vi "Find Outline.vi"(6 "Mask Info":i8[][](array[numeric]), 7 "Data":u8[][](array[numeric]), 8 "error in (no error)":errorcluster, 9 "Starting X (left)":i32, 10 "Starting Y (top)":i32, 11 "Outline in":refnum<class "Outline.lvclass">) -> (0 "error out":errorcluster, 3 "Outline out":refnum<class "Outline.lvclass">, 4 "Mask Info out":i8[][](array[numeric]))   [LabVIEW 2013, in "Outline.lvclass"]
uses:
  Outline.lvclass
  Outline.lvclass/Outline.ctl
  <vilib>/vision/NI_Vision_Development_Module.lvlib
panel:
  out "Mask Info out 2":i8[][](array[numeric])
  out "Image 3":T1(plugin-control)
  out "Image 2":T1(plugin-control)
  in  "Maximum number of points":i32=1000
  out "XY Graph":cluster{"X Values":i32[], "Y Values":i32[]}(graph)
  out "Y Values":i32[](array[numeric])
  out "X Values":i32[](array[numeric])
  # "Top first, then left"
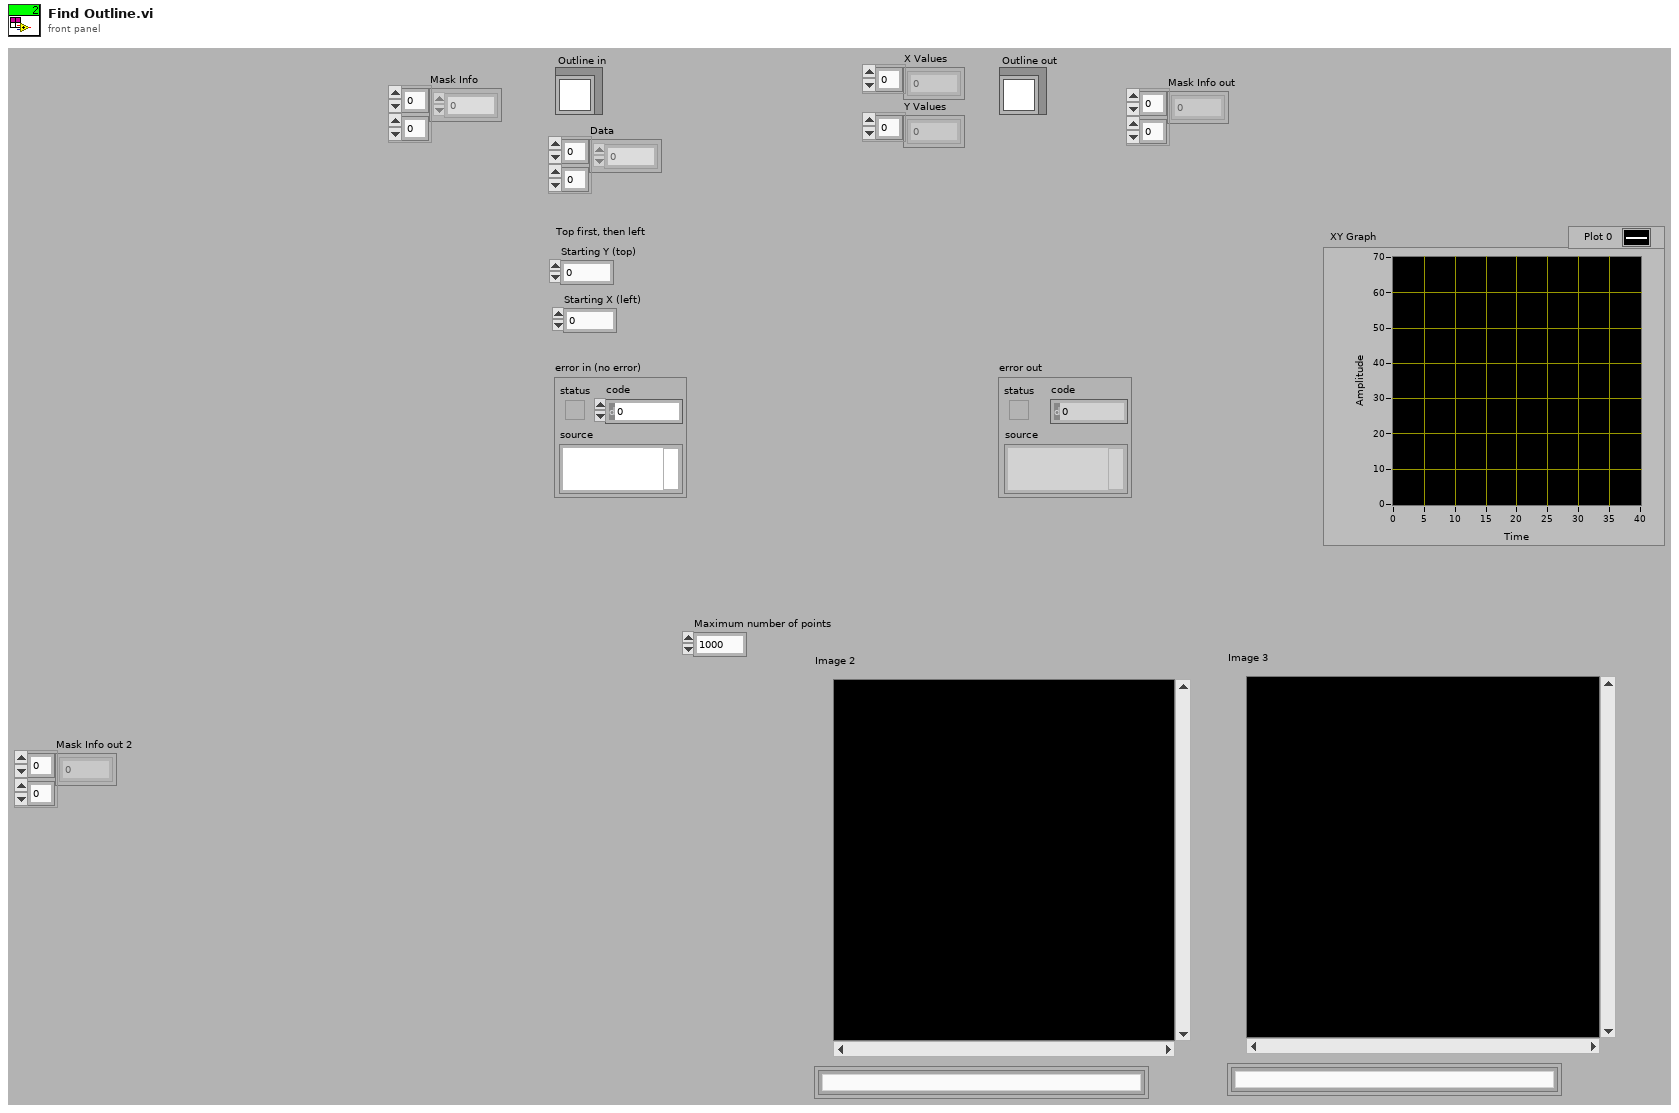
[diagram p1: front panel]
types:
  T1 = typedef "IMAQ Image.ctl" = refnum<image>
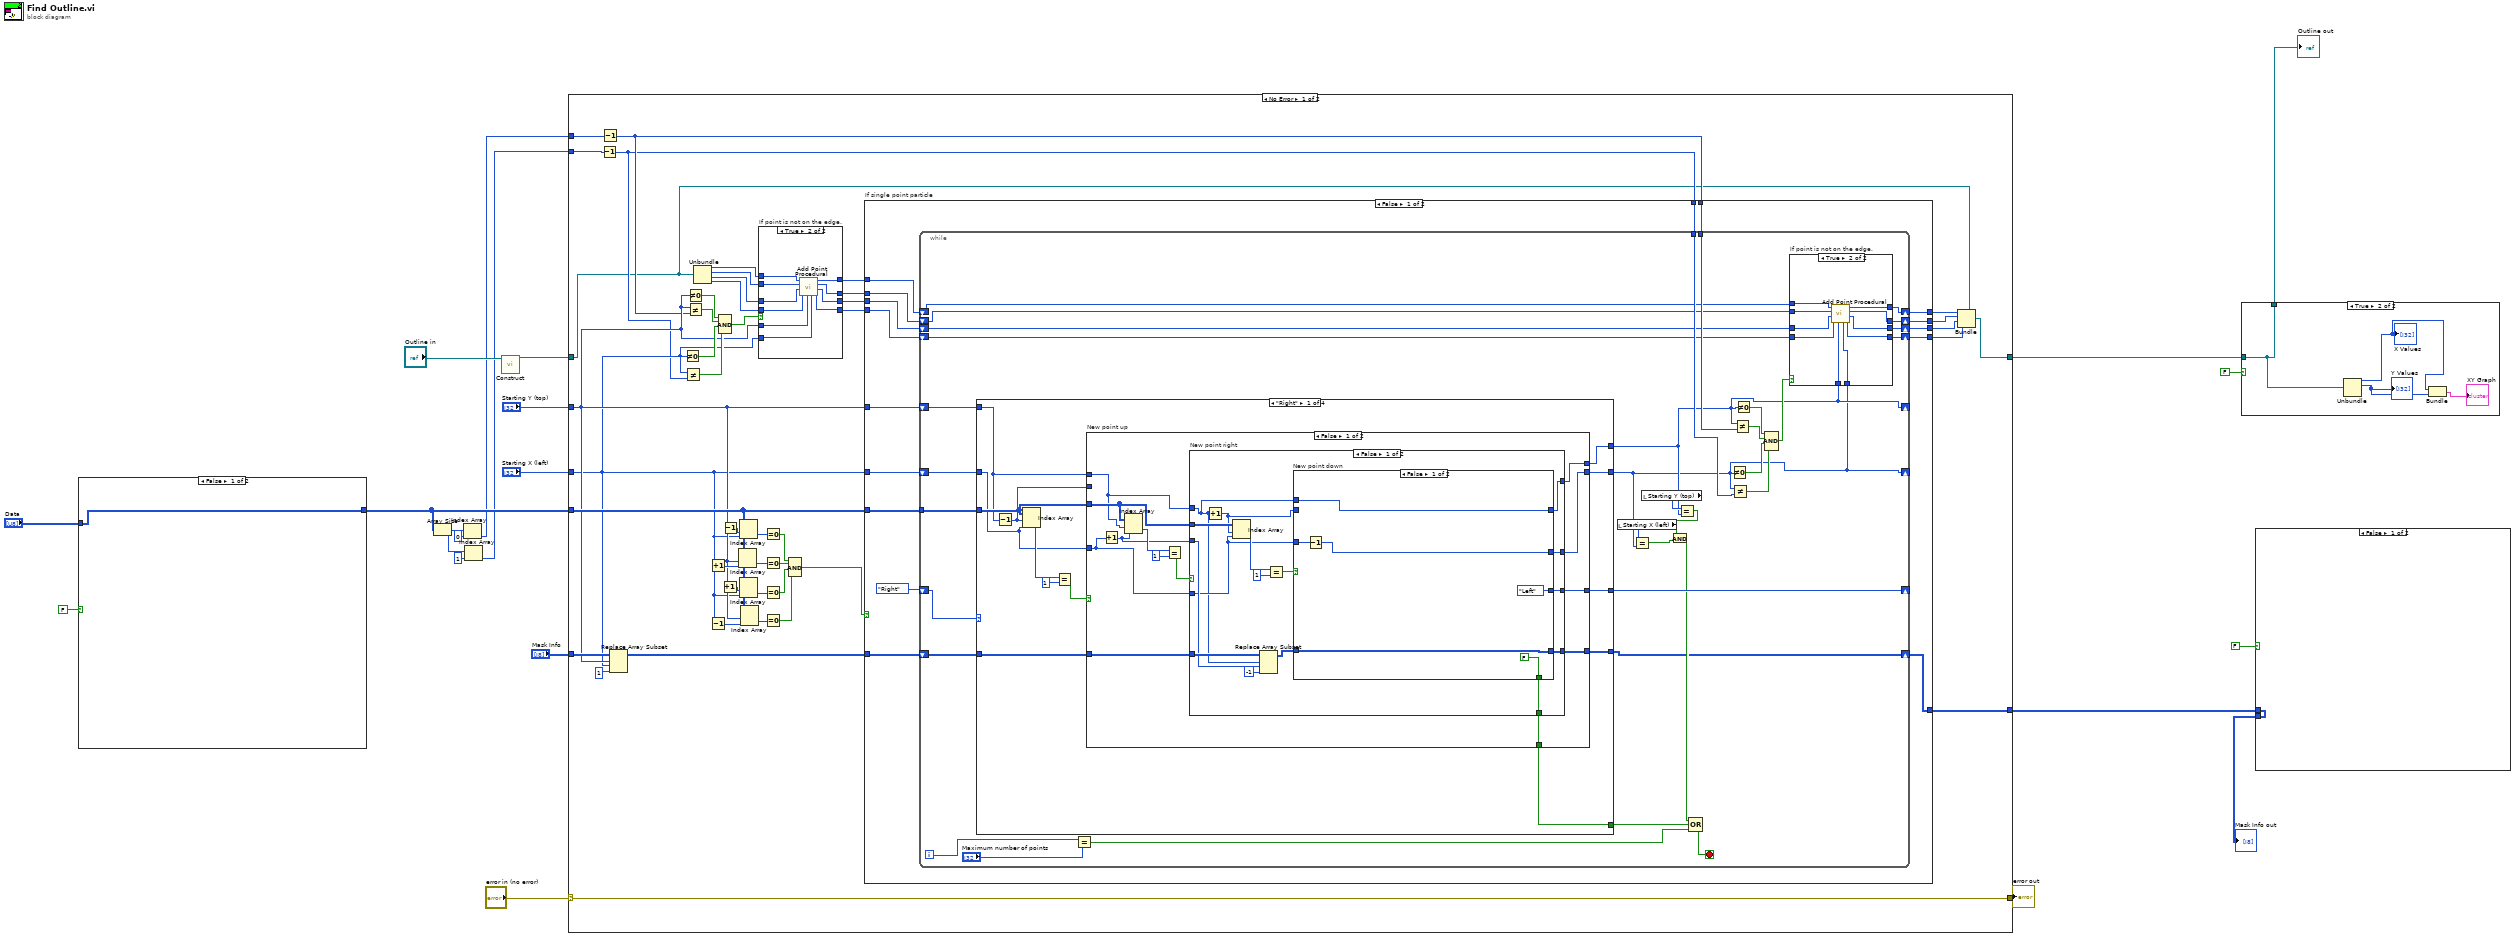
[diagram p0: block diagram]
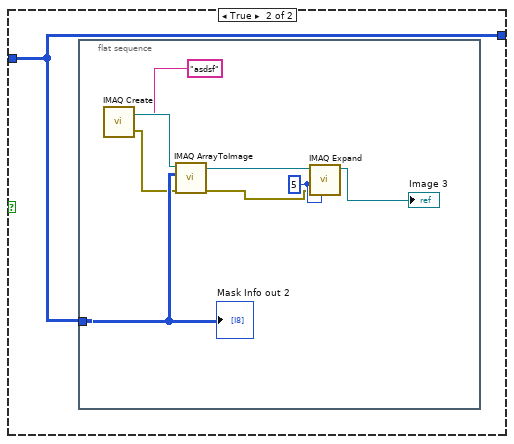
[diagram p2: hidden frame]
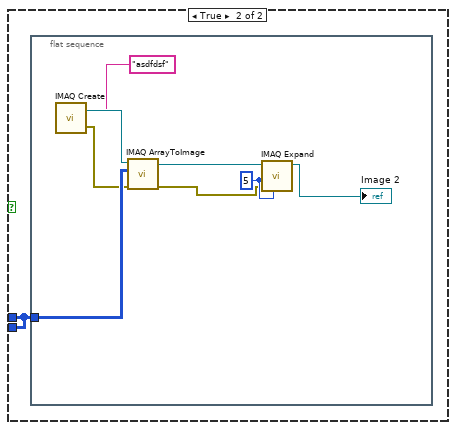
[diagram p3: hidden frame]
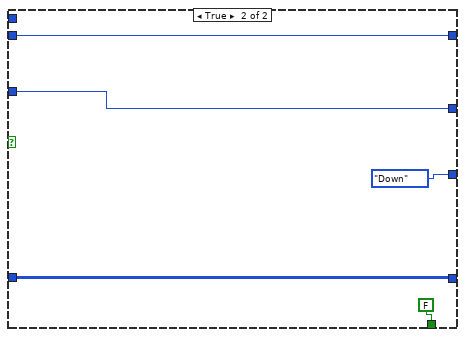
[diagram p7: hidden frame]
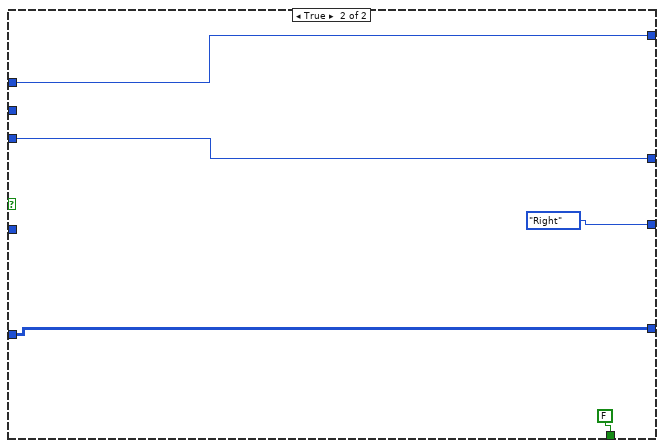
[diagram p8: hidden frame]
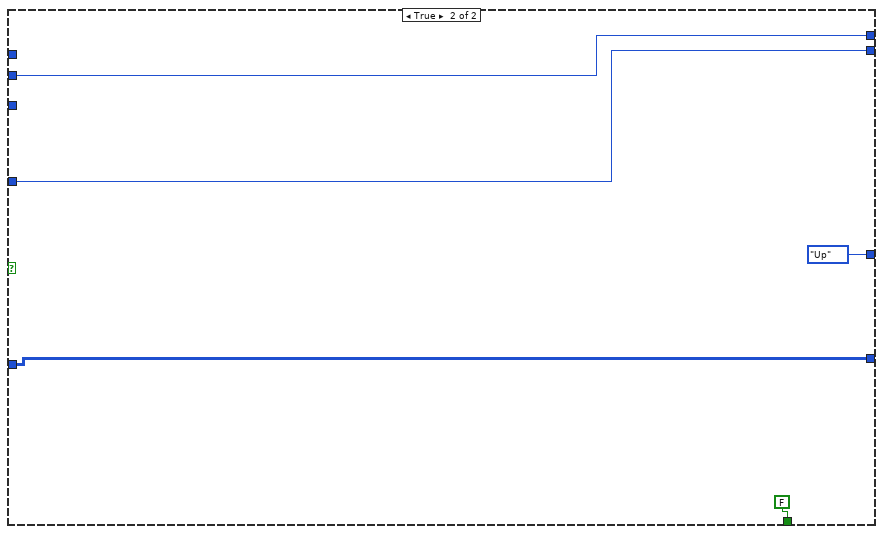
[diagram p9: hidden frame]
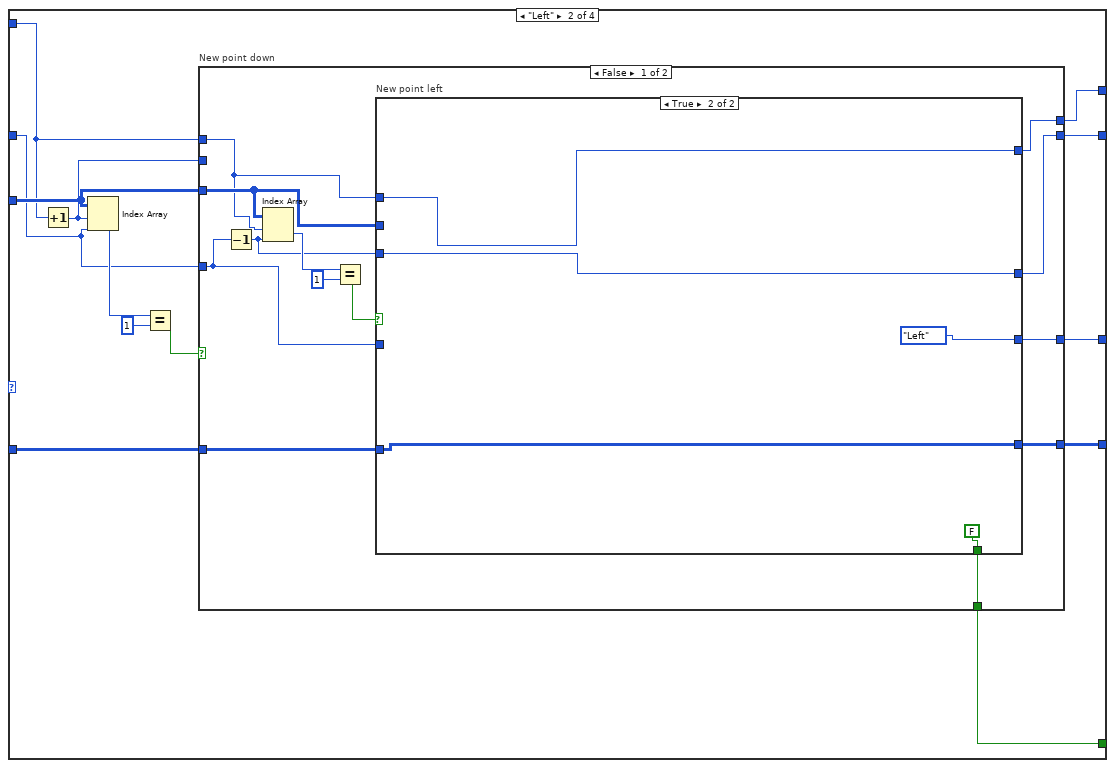
[diagram p10: hidden frame]
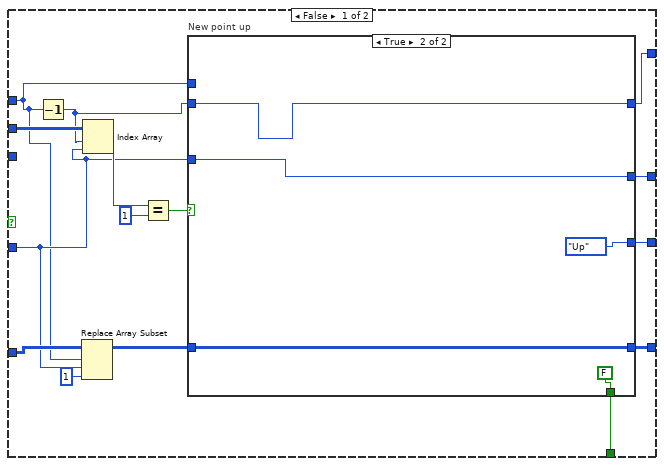
[diagram p11: hidden frame]
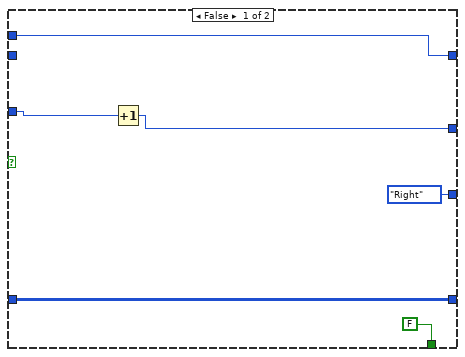
[diagram p12: hidden frame]
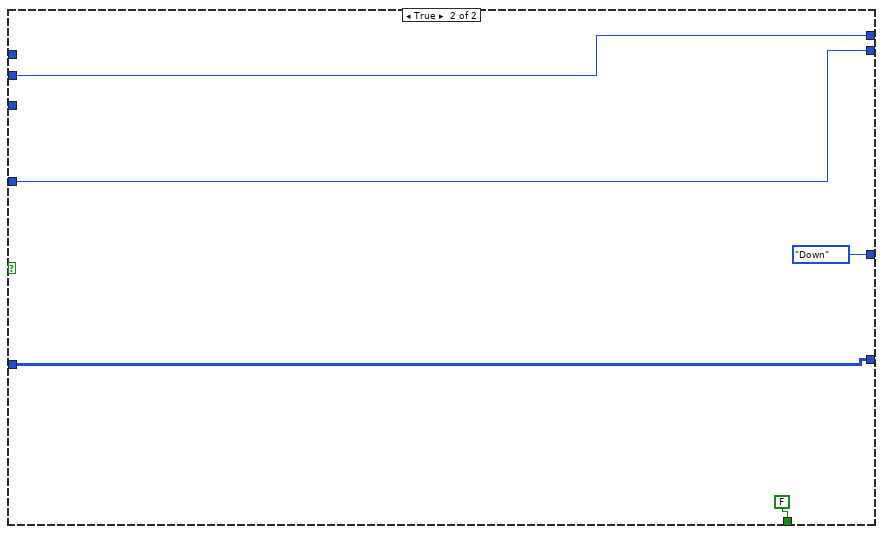
[diagram p13: hidden frame]
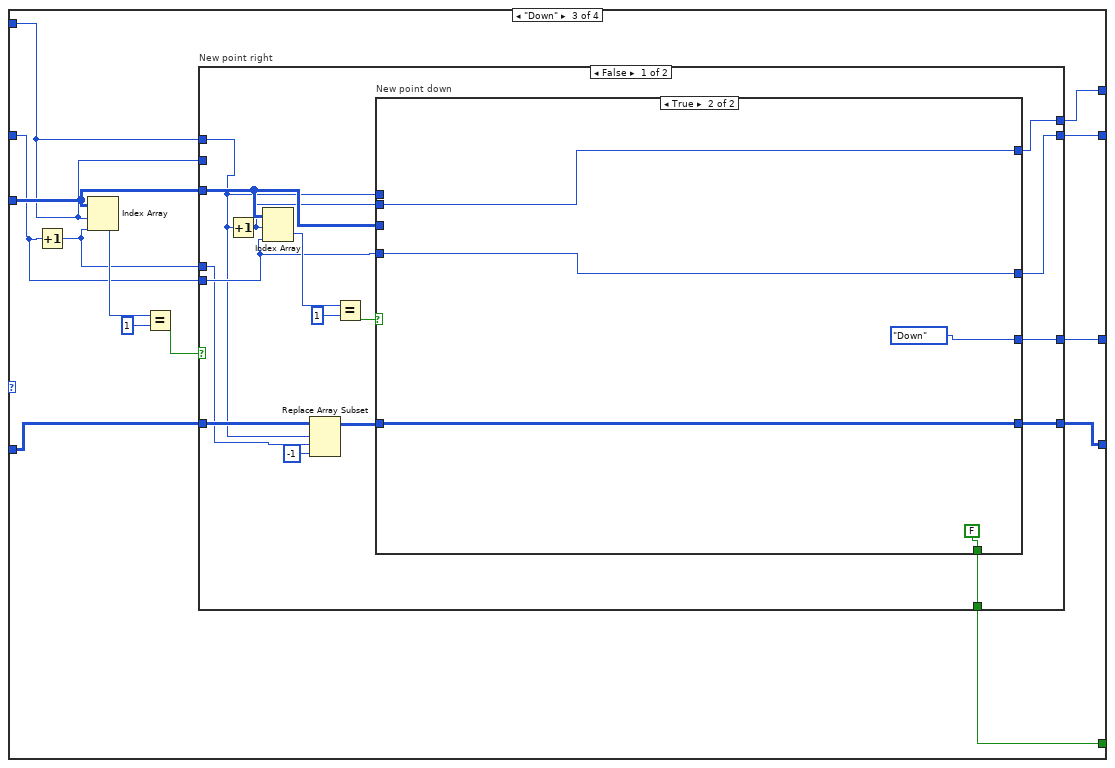
[diagram p14: hidden frame]
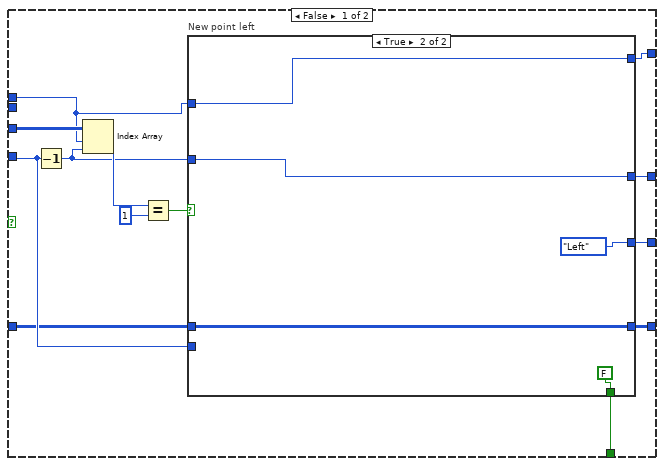
[diagram p15: hidden frame]
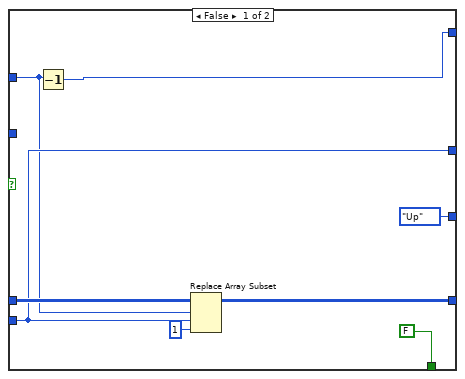
[diagram p16: hidden frame]
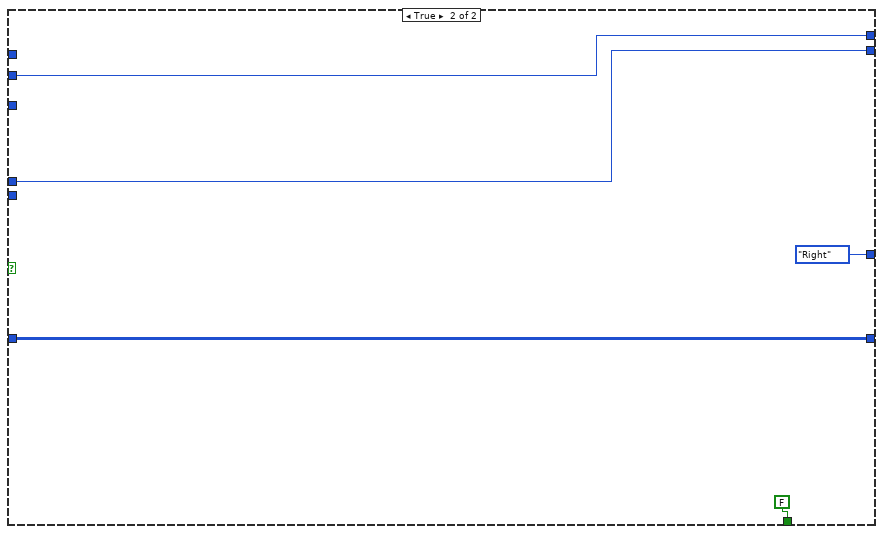
[diagram p17: hidden frame]
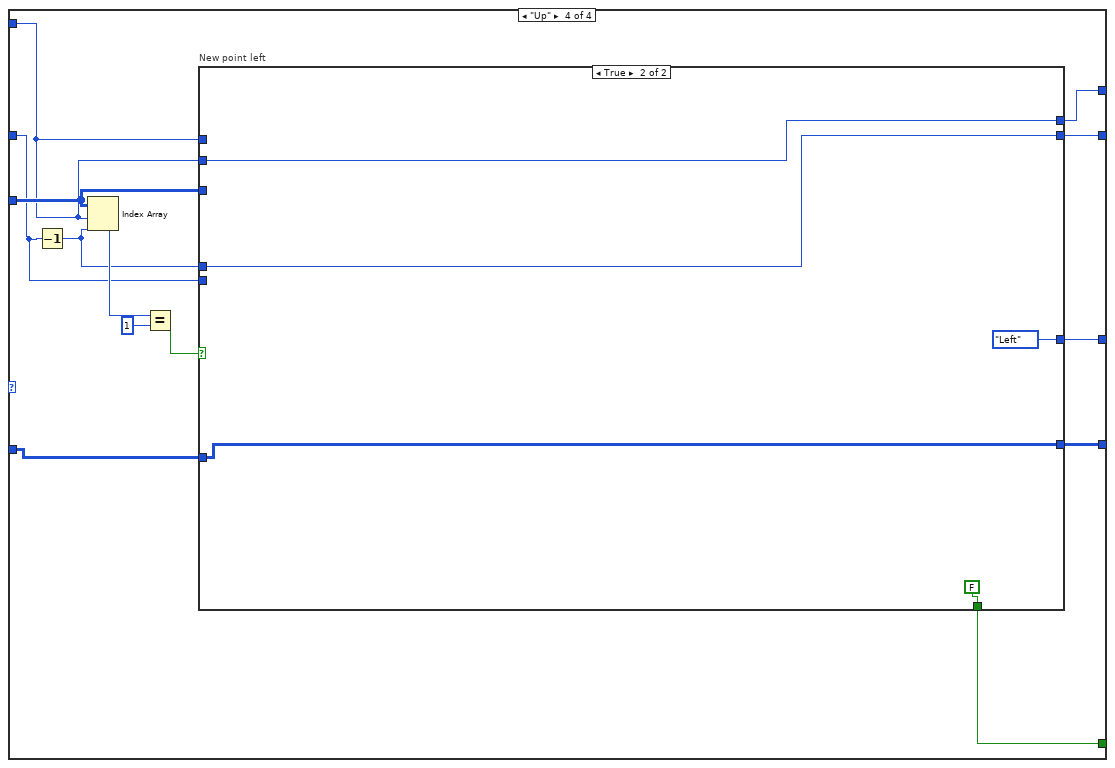
[diagram p18: hidden frame]
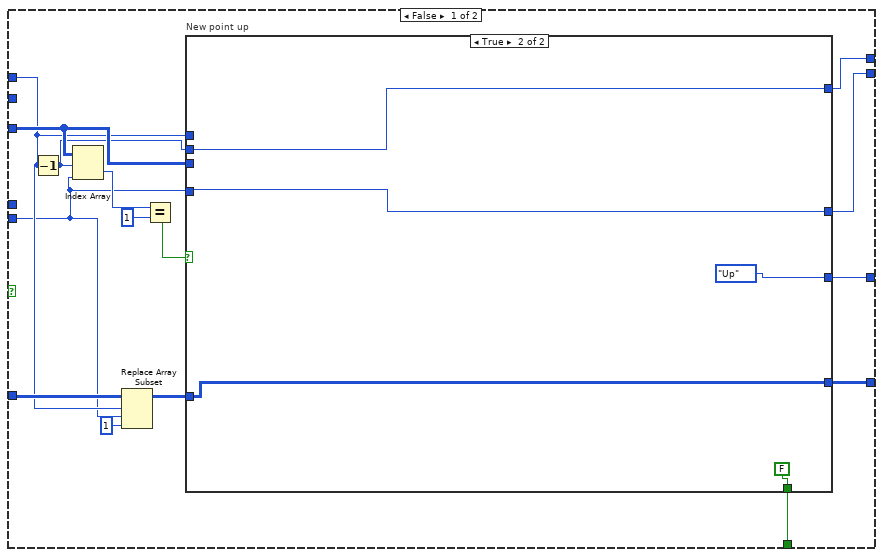
[diagram p19: hidden frame]
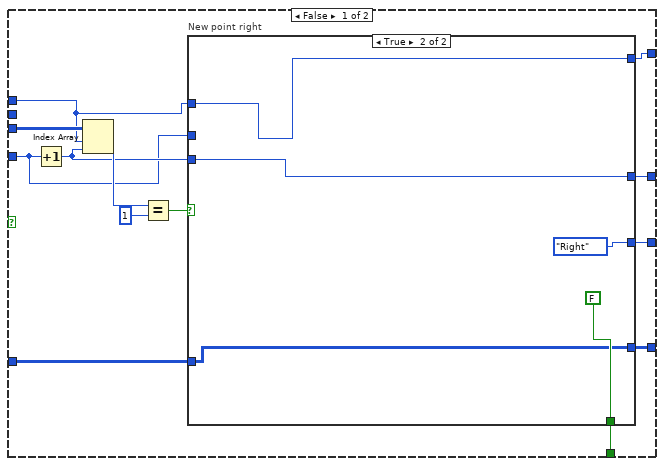
[diagram p20: hidden frame]
diagram:
  n1 = case shown="False" FALSE {
    tunnel: [w22 w23] -> w3
    tunnel: "Data" -> [w22 w23]
    frame False {
    }
    frame True {
      n2 = flat-sequence {
        tunnel: w23 -> [w30]
        frame #0 {
          w31 = 5 ("X Duplication Step")
          n3 = call "IMAQ Create"("Image Name"="asdsf") -> ("New Image"=w25:T1, "error out"=w26:errorcluster)  [unwired: 4 in]
          n4 = call "IMAQ ArrayToImage"("error in (no error)"=w26, "Image Pixels (U8)"=w30, "Image"=w25) -> ("error out"=w28:errorcluster, "Image Out"=w29:T1)  [unwired: 7 in]
          n5 = call "IMAQ Expand"("Y Duplication Step"=w31, "error in (no error)"=w28, "X Duplication Step"=w31, "Image Src"=w29) -> ("Image Dst Out"=→"Image 3":T1)  [unwired: 6 in, 1 out]
          "Mask Info out 2" <- w30
        }
      }
    }
  }
  n6 = Array Size(array=w3) -> (size(s)=w7:i32[])
  n7 = Index Array(array=w7, index=0) -> (element=w2:i32)
  n8 = Index Array(array=w7, index=1) -> (element=w1:i32)
  n9 = call-dynamic "Construct.vi"("Outline in"="Outline in") -> ("Outline out"=w17:refnum<class "Outline.lvclass">)  [unwired: 9 in, 1 out]
  n10 = case shown="No Error" "error in (no error)" {
    selector: "error in (no error)" -> [w75 w420]
    tunnel: [w75 w420] -> w21
    tunnel: [w32 w419] -> w20
    tunnel: w17 -> [w37 w419]
    tunnel: "Starting Y (top)" -> [w51 _]
    tunnel: "Starting X (left)" -> [w50 _]
    tunnel: w3 -> [w69 _]
    tunnel: "Mask Info" -> [w73 w418]
    tunnel: [w74 w418] -> w9
    tunnel: w2 -> [w41 _]
    tunnel: w1 -> [w39 _]
    frame No Error {
      n11 = Decrement(x=w39) -> (x-1=w38:i32)
      n12 = Decrement(x=w41) -> (x-1=w40:i32)
      n13 = Replace Array Subset(array=w73, new element=i8 1 ("new element/subarray"), index (row)=w51, index (col)=w50) -> (w72:i8[][])
      n14 = Not Equal To 0?(x=w50) -> (x != 0?=w54:bool)
      n15 = Not Equal?(x=w50, y=w38) -> (x != y?=w55:bool)
      n16 = Not Equal To 0?(x=w51) -> (x != 0?=w52:bool)
      n17 = Not Equal?(x=w51, y=w40) -> (x != y?=w53:bool)
      n18 = Unbundle(w37) -> (w49:i32[], w46:i32[], w47:i32, w48:i32)
      n19 = Increment(x=w50) -> (x+1=w68:i32)
      n20 = Decrement(x=w50) -> (x-1=w66:i32)
      n21 = Compound Arithmetic op=AND(w52, w53, w54, w55) -> (w56:bool)
      n22 = Increment(x=w51) -> (x+1=w67:i32)
      n23 = Decrement(x=w51) -> (x-1=w70:i32)
      n24 = Index Array(array=w69, index (row)=w51, index (col)=w68) -> (element=w64:u8)
      n25 = Index Array(array=w69, index (row)=w70, index (col)=w50) -> (element=w65:u8)
      n26 = Index Array(array=w69, index (row)=w67, index (col)=w50) -> (element=w63:u8)
      n27 = Index Array(array=w69, index (row)=w51, index (col)=w66) -> (element=w62:u8)
      n28 = case "If point is not on the edge." shown="True" w56 {
        tunnel: w51 -> [_ w89]
        tunnel: w50 -> [_ w88]
        tunnel: w49 -> [w79 w87]
        tunnel: w46 -> [w78 w86]
        tunnel: w47 -> [w77 w85]
        tunnel: w48 -> [w76 w84]
        tunnel: [w79 w83] -> w45
        tunnel: [w78 w82] -> w44
        tunnel: [w77 w81] -> w43
        tunnel: [w76 w80] -> w42
        frame False {
        }
        frame True {
          n29 = call "Add Point Procedural.vi"("New X"=w88, "New Y"=w89, "Memory allocated in"=w84, "Number of points in"=w85, "Y Values in"=w86, "X Values in"=w87) -> ("Memory allocated out"=w80:i32, "Number of Points out"=w81:i32, "Y Values out"=w82:i32[], "X Values out"=w83:i32[])  [unwired: 2 in]
        }
      }
      n30 = Equal To 0?(x=w65) -> (x = 0?=w61:bool)
      n31 = Equal To 0?(x=w64) -> (x = 0?=w60:bool)
      n32 = Equal To 0?(x=w63) -> (x = 0?=w59:bool)
      n33 = Equal To 0?(x=w62) -> (x = 0?=w58:bool)
      n34 = Compound Arithmetic op=AND(w61, w60, w59, w58) -> (w57:bool)
      n35 = case "If single point particle" shown="False" w57 {
        tunnel: [w104 w412] -> w74
        tunnel: w72 -> [w103 w417]
        tunnel: w69 -> [w102 _]
        tunnel: w50 -> [w101 w415]
        tunnel: w51 -> [w100 w416]
        tunnel: w40 -> [w99 _]
        tunnel: w38 -> [w98 _]
        tunnel: w45 -> [w97 w411]
        tunnel: w44 -> [w96 w410]
        tunnel: w43 -> [w95 w409]
        tunnel: w42 -> [w94 w408]
        tunnel: [w93 w411] -> w36
        tunnel: [w92 w410] -> w35
        tunnel: [w91 w409] -> w34
        tunnel: [w90 w408] -> w33
        frame False {
          n36 = while {
            shift-right: [w115] -> _
            shift-left: w100 -> [w138]
            shift-right: [w114] -> _
            shift-left: w101 -> [w137]
            shift-right: [w135] -> _
            shift-left: enum16{"Up", "Left", "Down", "Right"}."Right" ("Enum") -> [w139]
            tunnel: w102 -> [w136]
            shift-right: [w123] -> w104
            shift-left: w103 -> [w124]
            tunnel: w99 -> [w122]
            tunnel: w98 -> [w121]
            shift-right: [w109] -> w93
            shift-left: w97 -> [w113]
            shift-right: [w108] -> w92
            shift-left: w96 -> [w112]
            shift-right: [w107] -> w91
            shift-left: w95 -> [w111]
            shift-right: [w106] -> w90
            shift-left: w94 -> [w110]
            i -> [w127]
            stop <- w128 stop-if-true
            n37 = case shown="\"Right\"" w139 {
              tunnel: w138 -> [w156 w219 w283 w348]
              tunnel: w137 -> [w157 w220 w282 w347]
              tunnel: w136 -> [w160 w223 w285 w350]
              tunnel: [w166 w229 w291 w356] -> w135
              tunnel: [w165 w228 w290 w355] -> w115
              tunnel: [w164 w227 w289 w354] -> w114
              tunnel: [w159 w222 w284 w349] -> w130
              tunnel: w124 -> [w155 w218 w280 w345]
              tunnel: [w154 w217 w279 w344] -> w123
              frame "Right" {
                n38 = Decrement(x=w156) -> (x-1=w158:i32)
                n39 = Index Array(array=w160, index (row)=w158, index (col)=w157) -> (element=w163:u8)
                n40 = Equal?(x=w163, y=u8 1) -> (x = y?=w161:bool)
                n41 = case "New point up" shown="False" w161 {
                  tunnel: [w176 enum16{"Up", "Left", "Down", "Right"}."Up" ("Enum")] -> w166
                  tunnel: w158 -> [_ w214]
                  tunnel: w157 -> [w169 w215]
                  tunnel: [w175 w214] -> w165
                  tunnel: [w174 w215] -> w164
                  tunnel: w160 -> [w173 _]
                  tunnel: [w172 FALSE] -> w159
                  tunnel: w156 -> [w171 _]
                  tunnel: w155 -> [w168 w212]
                  tunnel: [w167 w212] -> w154
                  frame False {
                    n42 = Increment(x=w169) -> (x+1=w170:i32)
                    n43 = Index Array(array=w173, index (row)=w171, index (col)=w170) -> (element=w177:u8)
                    n44 = Equal?(x=w177, y=u8 1) -> (x = y?=w178:bool)
                    n45 = case "New point right" shown="False" w178 {
                      tunnel: w171 -> [w180 w210]
                      tunnel: w170 -> [w182 w209]
                      tunnel: [w195 enum16{"Up", "Left", "Down", "Right"}."Right" ("Enum")] -> w176
                      tunnel: [w189 w210] -> w175
                      tunnel: [w188 w209] -> w174
                      tunnel: w173 -> [w194 _]
                      tunnel: [w190 FALSE] -> w172
                      tunnel: w169 -> [w181 _]
                      tunnel: w168 -> [w186 w207]
                      tunnel: [w184 w207] -> w167
                      frame False {
                        n46 = Increment(x=w180) -> (x+1=w183:i32)
                        n47 = Index Array(array=w194, index (row)=w183, index (col)=w181) -> (element=w192:u8)
                        n48 = Replace Array Subset(array=w186, new element=i8 -1 ("new element/subarray"), index (row)=w180, index (col)=w182) -> (w185:i8[][])
                        n49 = Equal?(x=w192, y=u8 1) -> (x = y?=w191:bool)
                        n50 = case "New point down" shown="False" w191 {
                          tunnel: [enum16{"Up", "Left", "Down", "Right"}."Left" ("Enum") enum16{"Up", "Left", "Down", "Right"}."Down" ("Enum")] -> w195
                          tunnel: w183 -> [_ w204]
                          tunnel: w181 -> [w197 w203]
                          tunnel: [FALSE FALSE] -> w190
                          tunnel: [w198 w204] -> w189
                          tunnel: [w196 w203] -> w188
                          tunnel: [w199 w202] -> w184
                          tunnel: w185 -> [w199 w202]
                          tunnel: w180 -> [w198 _]
                          frame False {
                            n51 = Decrement(x=w197) -> (x-1=w196:i32)
                          }
                          frame True {
                          }
                        }
                      }
                      frame True {
                      }
                    }
                  }
                  frame True {
                  }
                }
              }
              frame "Left" {
                n52 = Increment(x=w219) -> (x+1=w221:i32)
                n53 = Index Array(array=w223, index (row)=w221, index (col)=w220) -> (element=w226:u8)
                n54 = Equal?(x=w226, y=u8 1) -> (x = y?=w224:bool)
                n55 = case "New point down" shown="False" w224 {
                  tunnel: [w239 enum16{"Up", "Left", "Down", "Right"}."Down" ("Enum")] -> w229
                  tunnel: w221 -> [_ w275]
                  tunnel: w220 -> [w232 w274]
                  tunnel: [w238 w275] -> w228
                  tunnel: [w237 w274] -> w227
                  tunnel: w223 -> [w236 _]
                  tunnel: [w235 FALSE] -> w222
                  tunnel: w219 -> [w234 _]
                  tunnel: w218 -> [w231 w276]
                  tunnel: [w230 w276] -> w217
                  frame False {
                    n56 = Decrement(x=w232) -> (x-1=w233:i32)
                    n57 = Index Array(array=w236, index (row)=w234, index (col)=w233) -> (element=w240:u8)
                    n58 = Equal?(x=w240, y=u8 1) -> (x = y?=w241:bool)
                    n59 = case "New point left" shown="True" w241 {
                      tunnel: w234 -> [w243 w272]
                      tunnel: w233 -> [_ w271]
                      tunnel: [w257 enum16{"Up", "Left", "Down", "Right"}."Left" ("Enum")] -> w239
                      tunnel: [w251 w272] -> w238
                      tunnel: [w250 w271] -> w237
                      tunnel: w236 -> [w256 _]
                      tunnel: [w252 FALSE] -> w235
                      tunnel: w232 -> [w247 _]
                      tunnel: w231 -> [w248 w269]
                      tunnel: [w244 w269] -> w230
                      frame False {
                        n60 = Decrement(x=w243) -> (x-1=w249:i32)
                        n61 = Replace Array Subset(array=w248, new element=i8 1 ("new element/subarray"), index (row)=w243, index (col)=w247) -> (w245:i8[][])
                        n62 = Index Array(array=w256, index (row)=w249, index (col)=w247) -> (element=w254:u8)
                        n63 = Equal?(x=w254, y=u8 1) -> (x = y?=w253:bool)
                        n64 = case "New point up" shown="True" w253 {
                          tunnel: [enum16{"Up", "Left", "Down", "Right"}."Right" ("Enum") enum16{"Up", "Left", "Down", "Right"}."Up" ("Enum")] -> w257
                          tunnel: w249 -> [_ w266]
                          tunnel: w247 -> [w260 w265]
                          tunnel: [FALSE FALSE] -> w252
                          tunnel: [w258 w266] -> w251
                          tunnel: [w259 w265] -> w250
                          tunnel: [w261 w264] -> w244
                          tunnel: w245 -> [w261 w264]
                          tunnel: w243 -> [w258 _]
                          frame False {
                            n65 = Increment(x=w260) -> (x+1=w259:i32)
                          }
                          frame True {
                          }
                        }
                      }
                      frame True {
                      }
                    }
                  }
                  frame True {
                  }
                }
              }
              frame "Down" {
                n66 = Increment(x=w282) -> (x+1=w281:i32)
                n67 = Index Array(array=w285, index (row)=w283, index (col)=w281) -> (element=w288:u8)
                n68 = Equal?(x=w288, y=u8 1) -> (x = y?=w286:bool)
                n69 = case "New point right" shown="False" w286 {
                  tunnel: [w304 enum16{"Up", "Left", "Down", "Right"}."Right" ("Enum")] -> w291
                  tunnel: w283 -> [_ w341]
                  tunnel: w281 -> [w292 w342]
                  tunnel: [w303 w341] -> w290
                  tunnel: [w302 w342] -> w289
                  tunnel: w285 -> [w301 _]
                  tunnel: [w300 FALSE] -> w284
                  tunnel: w283 -> [w293 _]
                  tunnel: w282 -> [w299 _]
                  tunnel: w280 -> [w295 w339]
                  tunnel: [w297 w339] -> w279
                  frame False {
                    n70 = Increment(x=w293) -> (x+1=w298:i32)
                    n71 = Index Array(array=w301, index (row)=w298, index (col)=w299) -> (element=w305:u8)
                    n72 = Replace Array Subset(array=w295, new element=i8 -1 ("new element/subarray"), index (row)=w293, index (col)=w292) -> (w294:i8[][])
                    n73 = Equal?(x=w305, y=u8 1) -> (x = y?=w306:bool)
                    n74 = case "New point down" shown="True" w306 {
                      tunnel: w293 -> [w312 _]
                      tunnel: w299 -> [w310 w337]
                      tunnel: [w320 enum16{"Up", "Left", "Down", "Right"}."Down" ("Enum")] -> w304
                      tunnel: [w314 w335] -> w303
                      tunnel: [w313 w337] -> w302
                      tunnel: w301 -> [w319 _]
                      tunnel: [w315 FALSE] -> w300
                      tunnel: w298 -> [_ w335]
                      tunnel: w294 -> [w309 w334]
                      tunnel: [w308 w334] -> w297
                      frame False {
                        n75 = Decrement(x=w310) -> (x-1=w311:i32)
                        n76 = Index Array(array=w319, index (row)=w312, index (col)=w311) -> (element=w317:u8)
                        n77 = Equal?(x=w317, y=u8 1) -> (x = y?=w316:bool)
                        n78 = case "New point left" shown="True" w316 {
                          tunnel: [enum16{"Up", "Left", "Down", "Right"}."Up" ("Enum") enum16{"Up", "Left", "Down", "Right"}."Left" ("Enum")] -> w320
                          tunnel: w312 -> [w321 w331]
                          tunnel: w311 -> [_ w330]
                          tunnel: [FALSE FALSE] -> w315
                          tunnel: [w322 w331] -> w314
                          tunnel: [w323 w330] -> w313
                          tunnel: w310 -> [w323 _]
                          tunnel: w309 -> [w325 w329]
                          tunnel: [w324 w329] -> w308
                          frame False {
                            n79 = Decrement(x=w321) -> (x-1=w322:i32)
                            n80 = Replace Array Subset(array=w325, new element=i8 1 ("new element/subarray"), index (row)=w321, index (col)=w323) -> (w324:i8[][])
                          }
                          frame True {
                          }
                        }
                      }
                      frame True {
                      }
                    }
                  }
                  frame True {
                  }
                }
              }
              frame "Up" {
                n81 = Decrement(x=w347) -> (x-1=w346:i32)
                n82 = Index Array(array=w350, index (row)=w348, index (col)=w346) -> (element=w353:u8)
                n83 = Equal?(x=w353, y=u8 1) -> (x = y?=w351:bool)
                n84 = case "New point left" shown="True" w351 {
                  tunnel: [w368 enum16{"Up", "Left", "Down", "Right"}."Left" ("Enum")] -> w356
                  tunnel: w348 -> [_ w405]
                  tunnel: w346 -> [_ w406]
                  tunnel: [w367 w405] -> w355
                  tunnel: [w366 w406] -> w354
                  tunnel: w350 -> [w365 _]
                  tunnel: [w364 FALSE] -> w349
                  tunnel: w348 -> [w358 _]
                  tunnel: w347 -> [w357 _]
                  tunnel: w345 -> [w361 w403]
                  tunnel: [w359 w403] -> w344
                  frame False {
                    n85 = Decrement(x=w358) -> (x-1=w363:i32)
                    n86 = Index Array(array=w365, index (row)=w363, index (col)=w357) -> (element=w369:u8)
                    n87 = Replace Array Subset(array=w361, new element=i8 1 ("new element/subarray"), index (row)=w358, index (col)=w357) -> (w360:i8[][])
                    n88 = Equal?(x=w369, y=u8 1) -> (x = y?=w370:bool)
                    n89 = case "New point up" shown="True" w370 {
                      tunnel: w358 -> [w376 _]
                      tunnel: w357 -> [w372 w400]
                      tunnel: [w384 enum16{"Up", "Left", "Down", "Right"}."Up" ("Enum")] -> w368
                      tunnel: [w378 w399] -> w367
                      tunnel: [w377 w400] -> w366
                      tunnel: w365 -> [w383 _]
                      tunnel: [w379 FALSE] -> w364
                      tunnel: w363 -> [_ w399]
                      tunnel: w360 -> [w374 w398]
                      tunnel: [w373 w398] -> w359
                      frame False {
                        n90 = Increment(x=w372) -> (x+1=w375:i32)
                        n91 = Index Array(array=w383, index (row)=w376, index (col)=w375) -> (element=w381:u8)
                        n92 = Equal?(x=w381, y=u8 1) -> (x = y?=w380:bool)
                        n93 = case "New point right" shown="True" w380 {
                          tunnel: [enum16{"Up", "Left", "Down", "Right"}."Down" ("Enum") enum16{"Up", "Left", "Down", "Right"}."Right" ("Enum")] -> w384
                          tunnel: w376 -> [w385 w395]
                          tunnel: w375 -> [w387 w394]
                          tunnel: [FALSE FALSE] -> w379
                          tunnel: [w386 w395] -> w378
                          tunnel: [w387 w394] -> w377
                          tunnel: w374 -> [w389 w393]
                          tunnel: [w388 w393] -> w373
                          tunnel: w372 -> [_ _]
                          frame False {
                            n94 = Increment(x=w385) -> (x+1=w386:i32)
                            n95 = Replace Array Subset(array=w389, new element=i8 -1 ("new element/subarray"), index (row)=w385, index (col)=w387) -> (w388:i8[][])
                          }
                          frame True {
                          }
                        }
                      }
                      frame True {
                      }
                    }
                  }
                  frame True {
                  }
                }
              }
            }
            n96 = Equal?(x=w127, y="Maximum number of points") -> (x = y?=w126:bool)
            n97 = local read "Starting X (left)"() -> (w134:i32)
            n98 = Equal?(x=w134, y=w114) -> (x = y?=w132:bool)
            n99 = local read "Starting Y (top)"() -> (w133:i32)
            n100 = Equal?(x=w133, y=w115) -> (x = y?=w131:bool)
            n101 = And(x=w131, y=w132) -> (x .and. y?=w129:bool)
            n102 = Compound Arithmetic op=OR(w129, w130, w126) -> (w128:bool)
            n103 = Not Equal To 0?(x=w114) -> (x != 0?=w118:bool)
            n104 = Not Equal?(x=w114, y=w121) -> (x != y?=w117:bool)
            n105 = Not Equal?(x=w115, y=w122) -> (x != y?=w119:bool)
            n106 = Not Equal To 0?(x=w115) -> (x != 0?=w120:bool)
            n107 = Compound Arithmetic op=AND(w120, w119, w118, w117) -> (w116:bool)
            n108 = case "If point is not on the edge." shown="True" w116 {
              tunnel: w115 -> [_ w153]
              tunnel: w114 -> [_ w152]
              tunnel: w113 -> [w143 w151]
              tunnel: w112 -> [w142 w150]
              tunnel: w111 -> [w141 w149]
              tunnel: w110 -> [w140 w148]
              tunnel: [w143 w147] -> w109
              tunnel: [w142 w146] -> w108
              tunnel: [w141 w145] -> w107
              tunnel: [w140 w144] -> w106
              frame False {
              }
              frame True {
                n109 = call "Add Point Procedural.vi"("New X"=w152, "New Y"=w153, "Memory allocated in"=w148, "Number of points in"=w149, "Y Values in"=w150, "X Values in"=w151) -> ("Memory allocated out"=w144:i32, "Number of Points out"=w145:i32, "Y Values out"=w146:i32[], "X Values out"=w147:i32[])  [unwired: 2 in]
              }
            }
          }
        }
        frame True {
          n110 = Increment(x=w415) -> (x+1=w414:i32)
          n111 = Replace Array Subset(array=w417, new element=i8 -1 ("new element/subarray"), index (row)=w416, index (col)=w414) -> (w412:i8[][])
        }
      }
      n112 = Bundle(cluster=w37, w36, w35, w34, w33) -> (w32:refnum<class "Outline.lvclass">)
    }
    frame Error {
    }
  }
  "error out" <- w21
  n113 = case shown="True" FALSE {
    tunnel: w20 -> [w421 w422]
    tunnel: [w421 w422] -> w12
    frame False {
    }
    frame True {
      n114 = Unbundle(w422) -> (w424:i32[], w425:i32[])  [unwired: 2 out]
      "X Values" <- w424
      "Y Values" <- w425
      n115 = Bundle("X Values"=w424, "Y Values"=w425) -> (→"XY Graph":cluster{"X Values":i32[], "Y Values":i32[]})  [unwired: 1 in]
    }
  }
  "Outline out" <- w12
  n116 = case shown="False" FALSE {
    tunnel: w9 -> [w426 w427]
    tunnel: [w426 w427] -> w5
    frame False {
    }
    frame True {
      n117 = flat-sequence {
        tunnel: w427 -> [w434]
        frame #0 {
          w435 = 5 ("X Duplication Step")
          n118 = call "IMAQ Create"("Image Name"="asdfdsf") -> ("New Image"=w429:T1, "error out"=w430:errorcluster)  [unwired: 4 in]
          n119 = call "IMAQ ArrayToImage"("error in (no error)"=w430, "Image Pixels (U8)"=w434, "Image"=w429) -> ("error out"=w432:errorcluster, "Image Out"=w433:T1)  [unwired: 7 in]
          n120 = call "IMAQ Expand"("Y Duplication Step"=w435, "error in (no error)"=w432, "X Duplication Step"=w435, "Image Src"=w433) -> ("Image Dst Out"=→"Image 2":T1)  [unwired: 6 in, 1 out]
        }
      }
    }
  }
  "Mask Info out" <- w5
